vi "Checku8.vi"(7 "Name":string, 11 "Red":T1) -> (1 "image":u8[](array[numeric]), 3 "Success":bool)   [LabVIEW 2019]
uses:
  <vilib>/picture/picture.llb/imagedata.ctl
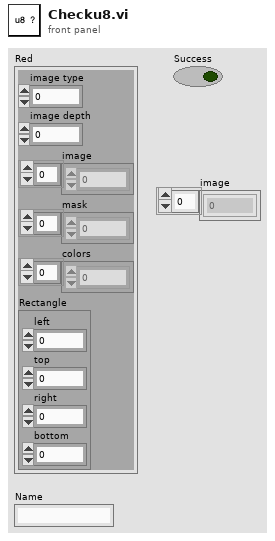
[diagram p1: front panel]
types:
  T1 = typedef "imagedata.ctl" = cluster{"image type":i32, "image depth":i32, "image":u8[], "mask":u8[], "colors":u32[], "Rectangle":cluster{"left":i16, "top":i16, "right":i16, "bottom":i16}}
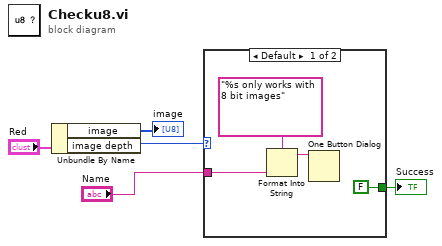
[diagram p0: block diagram]
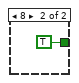
[diagram p2: hidden frame]
diagram:
  n1 = Unbundle By Name("Red") -> ("image"=→"image":u8[], "image depth"=w3:i32)
  n2 = case shown="Default" w3 {
    tunnel: "Name" -> [w8 _]
    tunnel: [FALSE TRUE] -> w5
    frame Default {
      n3 = Format Into String(format string="%s only works with 8 bit images" ("message"), w8) -> (resulting string=w6:string)  [unwired: 2 in, 1 out]
      n4 = One Button Dialog(message=w6) -> ()  [unwired: 1 in, 1 out]
    }
    frame 8 {
    }
  }
  "Success" <- w5
